vi "my_std_dev.vi"(8 "x 2":dbl[](array[numeric]), 11 "x":dbl[](array[numeric])) -> (2 "sqrt(x)":dbl[](array[numeric]))   [LabVIEW 2021, in "CALIBRATION.lvlib"]
uses:
  CALIBRATION.lvlib
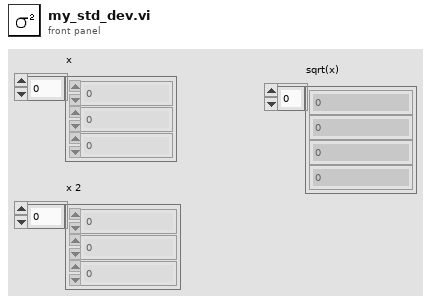
[diagram p1: front panel]
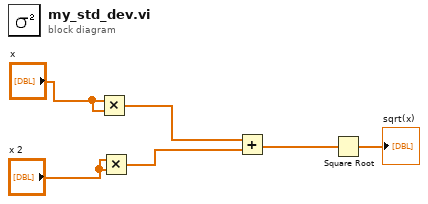
[diagram p0: block diagram]
diagram:
  n1 = Multiply(x="x", y="x") -> (x*y=w1:dbl[])
  n2 = Multiply(x="x 2", y="x 2") -> (x*y=w2:dbl[])
  n3 = Add(x=w1, y=w2) -> (x+y=w6:dbl[])
  n4 = Square Root(x=w6) -> (sqrt(x)=→"sqrt(x)":dbl[])
